vi "MVT_Query.vi"(0 "System no.":i32=1 min=1 max=4 step=1, 2 "Axes to query":string[](array[string]), 3 "All axes?":bool, 4 "Axis identifier?":bool=TRUE, 5 "error in":errorcluster) -> (14 "MVT trigger mode?":bool[](array[boolean]), 19 "error out":errorcluster)   [LabVIEW 2020]
doc: "Returns MVT trigger mode of queried axes.\n\nE-816: If All axes? = TRUE, then Axis identifier? can be FALSE. Check controller manual to find out if MVT? is supported."
panel:
  # "Returns MVT trigger mode of queried axes."
  # "If all axes: use"
  # "Query"
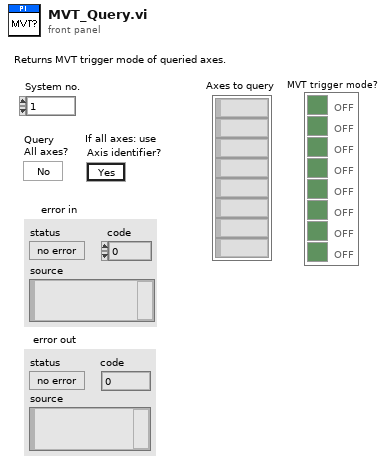
[diagram p1: front panel]
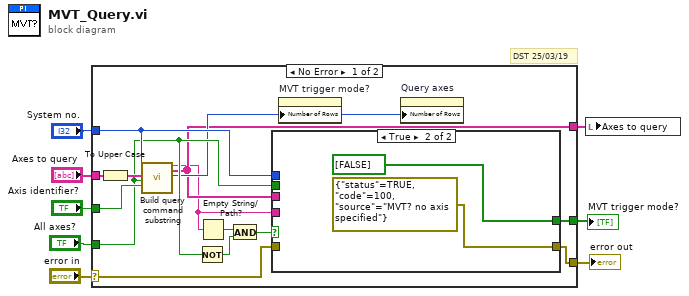
[diagram p0: block diagram]
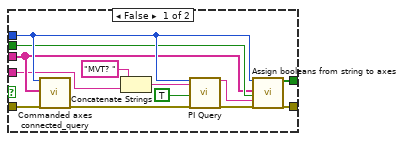
[diagram p2: hidden frame]
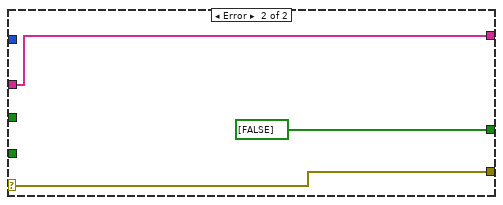
[diagram p3: hidden frame]
diagram:
  # "DST 25/03/19"
  n1 = case shown="No Error" "error in" {
    selector: "error in" -> [w9 w39]
    tunnel: [w22 bool[] [FALSE] ("Booleans")] -> w8
    tunnel: "Axes to query" -> [w21 w38]
    tunnel: [w20 w39] -> w6
    tunnel: "Axis identifier?" -> [w18 _]
    tunnel: "System no." -> [w17 _]
    tunnel: "All axes?" -> [w16 _]
    tunnel: [w13 w38] -> w2
    frame No Error {
      n2 = To Upper Case(1:w21) -> (0:w19:string[])
      n3 = call "Build query command substring.vi"("System no."=w17, "Axes to query in"=w19, "Query\nAll axes?"=w16, "For all axes: use\nAxis identifier?"=w18) -> ("Command substring"=w11:string, "Axes to query out"=w13:string[], "Number of rows"=w14:u32)  [unwired: 2 in, 11 out]
      n4 = Not(x=w16) -> (.not. x?=w15:bool)
      n5 = Empty String/Path?(string/path=w11) -> (empty?=w10:bool)
      n6 = And(x=w10, y=w15) -> (x .and. y?=w12:bool)
      n7 = case shown="True" w12 {
        tunnel: [w32 bool[] [FALSE] ("Booleans")] -> w22
        tunnel: w9 -> [w31 _]
        tunnel: [w28 errorcluster {"status"=TRUE, "code"=100, "source"="MVT? no axis specified"} ("error out")] -> w20
        tunnel: w11 -> [w23 _]
        tunnel: w17 -> [w30 _]
        tunnel: w16 -> [w29 _]
        tunnel: w13 -> [w24 _]
        frame False {
          n8 = call "Commanded axes connected_query.vi"("System no."=w30, "Commanded axes"=w24, "error in"=w31) -> ("error out"=w27:errorcluster)  [unwired: 1 in, 15 out]
          n9 = Concatenate Strings("MVT? ", w23) -> (w33:string)
          n10 = call "PI Query.vi"("System no."=w30, "String to send"=w33, "Attach termination char.?"=TRUE ("Attach Linefeed?"), "error in"=w27) -> ("String read"=w25:string, "error out"=w26:errorcluster)  [unwired: 3 in, 11 out]
          n11 = call "Assign booleans from string to axes.vi"("System no."=w30, "Queried axes"=w24, "All axes queried?"=w29, "Input String"=w25, "error in"=w26) -> ("Booleans"=w32:bool[], "error out"=w28:errorcluster)  [unwired: 13 out]
        }
        frame True {
        }
      }
      n12 = property on="MVT trigger mode?" class="Arr (strict)"("Number of Rows"=w14) -> ()  [unwired: 2 in, 2 out]
      n13 = property on="Query axes" class="Arr (strict)"("Number of Rows"=w14) -> ()  [unwired: 2 in, 2 out]
    }
    frame Error {
    }
  }
  "error out" <- w6
  "MVT trigger mode?" <- w8
  n14 = local write "Axes to query"(w2) -> ()
